vi "Constructor.vi"(5 "TimeZoneInfoId":string, 6 "SequenceExecutionStatus":T1=enum."NOT_COMPLETED", 7 "StartDate":timestamp, 8 "error in":errorcluster, 9 "StationFullName":string, 10 "SequenceFullName":string, 11 "Name":string) -> (0 "error out":errorcluster, 3 "SequenceRun out":refnum<class "SequenceRun.lvclass">)   [LabVIEW 2021, in "ProligentXMLGenerator.lvlib" / "SequenceRun.lvclass"]
uses:
  SequenceRun.lvclass
  SequenceRun.lvclass/SequenceRun.ctl
  Base/DateTime/DateTime.lvclass
  Base/ExecutionStatus/ExecutionStatus.lvclass
  Base/FullName/FullName.lvclass
  StepRun/StepRun/StepRun.lvclass
  Base/SequenceFullName/SequenceFullName.lvclass
  Data.ctl
  Base/NonEmptyString_255/NonEmptyString_255.lvclass
  Base/NonEmptyString_64/NonEmptyString_64.lvclass
  Base/Guid/Guid.lvclass
  Model/CustomData/CustomData.lvclass
  Failure/FailureReference/FailureReference.lvclass
  Model/Document/Document.lvclass
  Model/Characteristic/Characteristic.lvclass
  Base/ExecutionStatus/Value.ctl
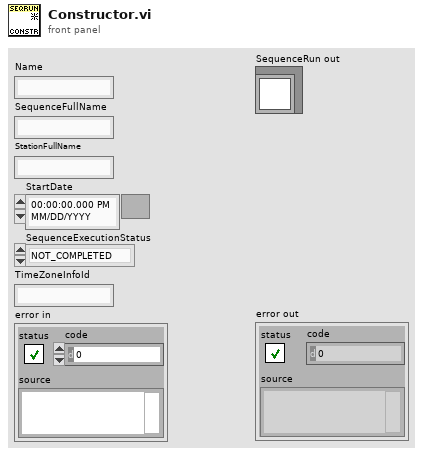
[diagram p1: front panel]
types:
  T1 = typedef "ProligentXMLGenerator.lvlib/ExecutionStatus.lvclass/Value.ctl" = enum16{"PASS", "FAIL", "NOT_COMPLETED", "ABORTED"}
  T2 = typedef "ProligentXMLGenerator.lvlib/SequenceRun.lvclass/Data.ctl" = cluster{"Name":string, "StepRuns":refnum<class "StepRun.lvclass">[], "Characteristics":refnum<class "Characteristic.lvclass">[], "Documents":refnum<class "Document.lvclass">[], "FailureReferences":refnum<class "FailureReference.lvclass">[], "CustomData":refnum<class "CustomData.lvclass">, "StartDate":refnum<class "DateTime.lvclass">, "EndDate":refnum<class "DateTime.lvclass">, "SequenceExecutionStatus":refnum<class "ExecutionStatus.lvclass">, "SequenceRunId":refnum<class "Guid.lvclass">, "SequenceFullName":refnum<class "SequenceFullName.lvclass">, "SequenceVersion":refnum<class "NonEmptyString_64.lvclass">, "StationFullName":refnum<class "FullName.lvclass">, "User":refnum<class "NonEmptyString_255.lvclass">, "TimeZoneInfoId":string}
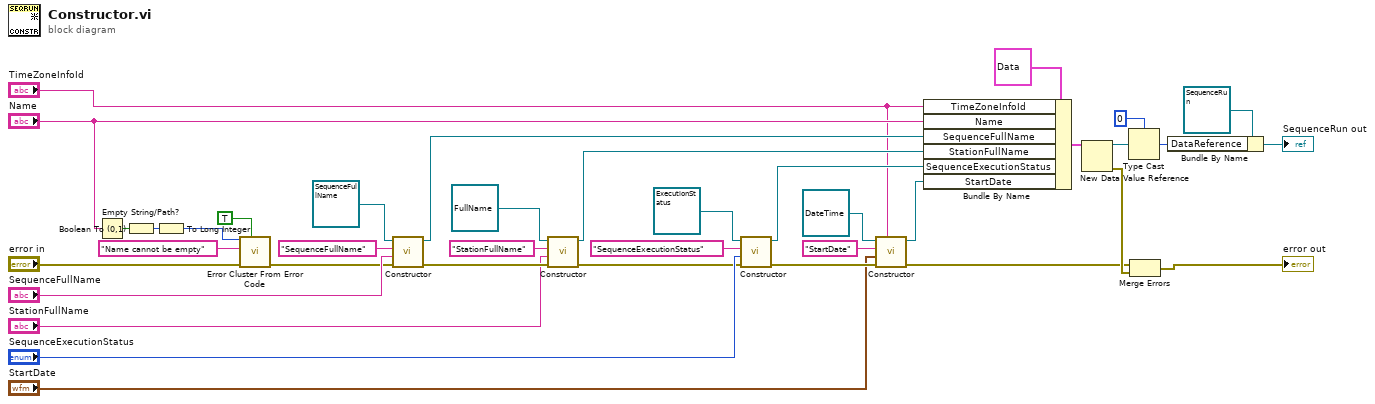
[diagram p0: block diagram]
diagram:
  n1 = Empty String/Path?(string/path="Name") -> (empty?=w23:bool)
  n2 = Boolean To (0,1)(Boolean=w23) -> (0, 1=w22:i16)
  n3 = To Long Integer(number=w22) -> (32bit integer=w21:i32)
  n4 = call <vilib>:"Error Cluster From Error Code.vi"("show call chain? (False)"=TRUE, "error in (no error)"="error in", "error message (\"\")"="Name cannot be empty" ("error message (\"\")"), "error code (0)"=w21) -> ("error out"=w19:errorcluster)  [unwired: 5 in]
  n5 = call-dynamic "Constructor.vi"("error in"=w19, "Value"="SequenceFullName", "Name"="SequenceFullName", "String in"=refnum<class "SequenceFullName.lvclass"> refnum ("ProligentResultProcessor:SequenceFullName")) -> ("error out"=w9:errorcluster, "String out"=w16:refnum<class "SequenceFullName.lvclass">)  [unwired: 6 in]
  n6 = call-dynamic "Constructor.vi"("error in"=w9, "Value"="StationFullName", "Name"="StationFullName", "String in"=refnum<class "FullName.lvclass"> refnum ("ProligentResultProcessor:NonEmptyString_65")) -> ("error out"=w8:errorcluster, "String out"=w7:refnum<class "FullName.lvclass">)  [unwired: 6 in]
  n7 = call-dynamic "Constructor.vi"("error in"=w8, "Value"="SequenceExecutionStatus", "Name"="SequenceExecutionStatus", "ExecutionStatus in"=refnum<class "ExecutionStatus.lvclass"> refnum ("ProligentResultProcessor:ExecutionStatus")) -> ("error out"=w15:errorcluster, "ExecutionStatus out"=w12:refnum<class "ExecutionStatus.lvclass">)  [unwired: 6 in]
  n8 = call-dynamic "Constructor.vi"("TimeZoneInfoId"="TimeZoneInfoId", "error in"=w15, "Value"="StartDate", "Name"="StartDate", "DateTime in"=refnum<class "DateTime.lvclass"> refnum) -> ("error out"=w18:errorcluster, "DateTime out"=w25:refnum<class "DateTime.lvclass">)  [unwired: 5 in]
  n9 = Bundle By Name(cluster=T2 {"Name"="", "StepRuns"=[], "Characteristics"=[], "Documents"=[], "FailureReferences"=[], "CustomData"=refnum, "StartDate"=refnum, "EndDate"=refnum, "SequenceExecutionStatus"=refnum, "SequenceRunId"=refnum, "SequenceFullName"=refnum, "SequenceVersion"=refnum, "StationFullName"=refnum, "User"=refnum, "TimeZoneInfoId"=""} ("Data"), "TimeZoneInfoId"="TimeZoneInfoId", "Name"="Name", "SequenceFullName"=w16, "StationFullName"=w7, "SequenceExecutionStatus"=w12, "StartDate"=w25) -> (w30:T2)
  n10 = New Data Value Reference(data value=w30) -> (data value reference=w29:refnum<data-value>, error out=w26:errorcluster)  [unwired: 1 in]
  n11 = Type Cast(type=u64 0, x=w29) -> (*(type *) &x=w27:u64)
  n12 = Merge Errors(w18, w26) -> (→"error out":errorcluster)
  n13 = Bundle By Name(cluster=refnum<class "SequenceRun.lvclass"> refnum ("ProligentResultProcessor:SequenceRun"), "DataReference"=w27) -> (→"SequenceRun out":refnum<class "SequenceRun.lvclass">)
